vi "Analyze.vi"(8 "error in (no error)":errorcluster, 10 "Image in":T1, 11 "Analyze SHG-AK in":refnum<class "Analyze SHG-AK.lvclass">) -> (0 "error out":errorcluster, 1 "Result":refnum<class "Analyze Results Base.lvclass">, 2 "Image out":T1, 3 "Analyze SHG-AK out":refnum<class "Analyze SHG-AK.lvclass">)   [LabVIEW 2020, in "Analyze.lvlib" / "Analyze SHG-AK.lvclass"]
uses:
  Analyze SHG-AK.lvclass
  C:/POLARIS Programme/POLARIS-AS-3-Cams/Submodules/HIJ Vision/Analyze/Analyze Classes/Analyze BaseClass/Analyze BaseClass/Analyze BaseClass.lvclass
  <vilib>/vision/Image Controls.llb/IMAQ Image.ctl
  Results and Overlays/Results Base/Analyze Results Base.lvclass
  Results and Overlays/Results SHG-AK/Analyze Results SHG-AK.lvclass
  C:/POLARIS Programme/POLARIS-AS-3-Cams/Submodules/HIJ Vision/Analyze/Results and Overlays/Results Base/Analyze Results Base.lvclass
  Analyze Parameter/Analyze Perameter Temporal Calibration/Analyze Parameter Temporal Calibration.lvclass
  C:/POLARIS Programme/POLARIS-AS-3-Cams/Submodules/HIJ Vision/Analyze/Analyze Parameter/Analyze Parameter Base/Analyze Parameter Base.lvclass
  Analyze Parameter/Analyze Perameter Temporal Calibration/Analyze Parameter Temporal Calibration.lvclass/Analyze Parameter Temporal Calibration.ctl
  Results and Overlays/Results SHG-AK/Analyze Results SHG-AK.lvclass/Analyze Results SHG-AK.ctl
  Analyze Parameter/Analyze Perameter Temporal Calibration/Read fs_px.vi
  Results and Overlays/Results SHG-AK/Write Gaussian Fit.vi
  Results and Overlays/Results SHG-AK/Write FWHM .vi
  Results and Overlays/Results SHG-AK/Write X-Values.vi
  Results and Overlays/Results SHG-AK/Write FWHM Gaussfit.vi
  Results and Overlays/Results SHG-AK/Write Y-ROI Averages.vi
  Analyze BaseClass/Analyze BaseClass/Analyze BaseClass.lvclass
  <vilib>/vision/NI_Vision_Development_Module.lvlib
  <vilib>/Analysis/NI_AALPro.lvlib
  Utility/POLARIS Vision utility.lvlib
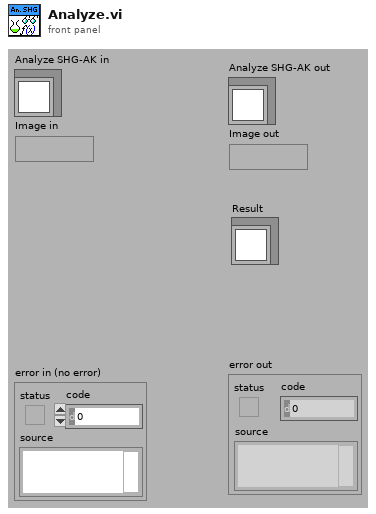
[diagram p1: front panel]
types:
  T1 = typedef "IMAQ Image.ctl" = refnum<image>
  T2 = typedef "ROI Descriptor" = cluster{"Global Rectangle":i32[], "Contours":cluster{"ID":enum32{"External", "Internal"}, "Type":u32, "Coordinates":i32[]}[]}
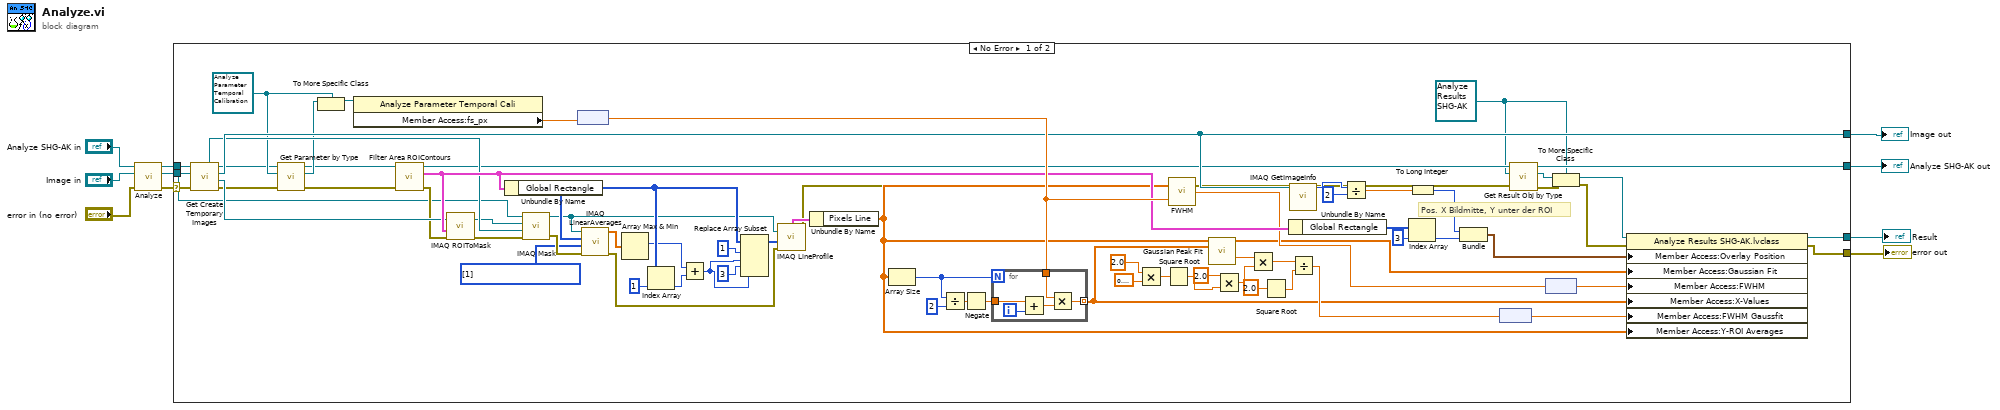
[diagram p0: block diagram]
diagram:
  n1 = call-parent "Analyze.vi"("error in (no error)"="error in (no error)", "Image in"="Image in", "Analyze BaseClass in"="Analyze SHG-AK in") -> ("error out"=w1:errorcluster, "Image out"=w5:T1, "Analyze BaseClass out"=w6:refnum<class "Analyze SHG-AK.lvclass">)  [unwired: 5 in, 1 out]
  n2 = case shown="No Error" w1 {
    selector: w1 -> [w19 w89]
    tunnel: [w67 w88] -> w10
    tunnel: w6 -> [w46 w90]
    tunnel: w5 -> [w45 w88]
    tunnel: [w28 _] -> w4
    tunnel: [w27 w89] -> w3
    tunnel: [w26 w90] -> w2
    frame No Error {
      w17 = refnum<class "Analyze Parameter Temporal Calibration.lvclass"> refnum ("Analyze Parameter Temporal Calibration.lvclass")
      w24 = refnum<class "Analyze Results SHG-AK.lvclass"> refnum ("Analyze Results SHG-AK.lvclass")
      w59 = i32[] [1] items=["X Axis Averages", "Y Axis Averages", "X + Y Axis Averages", "X - Y Axis Averages"] ("Averages")
      # "Pos. X Bildmitte, Y unter der ROI"
      n3 = call-dynamic "Get Create Temporary Images.vi"("error in (no error)"=w19, "Image in"=w45, "Analyze BaseClass in"=w46) -> ("error out"=w14:errorcluster, "image mask"=w65:T1, "work image"=w67:T1, "Analyze BaseClass out"=w15:refnum<class "Analyze SHG-AK.lvclass">, "masked image"=w64:T1)  [unwired: 4 in]
      n4 = call "Get Parameter by Type.vi"("error in (no error)"=w14, "Parameter Type"=w17, "Analyze BaseClass in"=w15) -> ("error out"=w13:errorcluster, "Parameter"=w18:refnum<class "Analyze Parameter Base.lvclass">, "Analyze BaseClass out"=w12:refnum<class "Analyze SHG-AK.lvclass">)  [unwired: 5 in, 1 out]
      n5 = To More Specific Class(target class=w17, reference=w18) -> (specific class reference=w16:refnum<class "Analyze Parameter Temporal Calibration.lvclass">)  [unwired: 1 in, 1 out]
      n6 = property class="Analyze Parameter Temporal Cali"(reference=w16) -> ("Member Access:fs_px"=w11:dbl[unit])  [unwired: 1 in, 2 out]
      n7 = call-dynamic "Filter Area ROIContours.vi"("error in (no error)"=w13, "Analyze BaseClass in"=w12) -> ("error out"=w61:errorcluster, "ROI of Area type"=w66:T2, "Analyze BaseClass out"=w29:refnum<class "Analyze SHG-AK.lvclass">)  [unwired: 7 in]
      n8 = call "IMAQ ROIToMask"("error in (no error)"=w61, "ROI Descriptor"=w66, "Image"=w65) -> ("error out"=w63:errorcluster, "Image Out"=w62:T1)  [unwired: 3 in, 1 out]
      n9 = Unbundle By Name(w66) -> ("Global Rectangle"=w55:i32[])
      n10 = call "IMAQ Mask"("error in (no error)"=w63, "Image Dst"=w64, "Image Mask"=w62, "Image Src"=w45) -> ("error out"=w60:errorcluster, "Image Dst Out"=w50:T1)  [unwired: 1 in]
      n11 = node(w11) -> (w82:dbl)
      n12 = call "IMAQ LinearAverages"("error in (no error)"=w60, "Averages"=w59, "Optional Rectangle"=w55, "Image Src"=w50) -> ("error out"=w48:errorcluster, "Y Axis Averages"=w58:sgl[])  [unwired: 3 in, 3 out]
      n13 = Array Max & Min(array=w58) -> (max index (indices)=w52:i32)  [unwired: 3 out]
      n14 = Index Array(array=w55, index=1) -> (element=w53:i32)
      n15 = Add(x=w52, y=w53) -> (x+y=w51:i32)
      n16 = Replace Array Subset(array=w55, new element #1=w51, index #1=1 ("index"), new element #2=w51, index #2=3 ("index")) -> (w49:i32[])
      n17 = call "IMAQ LineProfile"("error in (no error)"=w48, "Line Coordinates"=w49, "Image"=w50) -> ("error out"=w22:errorcluster, "Line Graph"=w47:cluster{"x0":sgl, "dx":sgl, "Pixels Line":sgl[]})  [unwired: 2 in, 2 out]
      n18 = Unbundle By Name(w47) -> ("Pixels Line"=w42:sgl[])
      n19 = Array Size(array=w42) -> (size(s)=w69:i32)
      n20 = Divide(x=w69, y=2) -> (x/y=w71:dbl)
      n21 = Negate(x=w71) -> (-x=w68:dbl)
      n22 = for {
        N: w69 -> [_]
        tunnel: w68 -> [w86]
        tunnel: [w84] -> w31 mode=indexing
        tunnel: w82 -> [w83]
        i -> [w87]
        n23 = Add(x=w86, y=w87) -> (x+y=w85:dbl)
        n24 = Multiply(x=w83, y=w85) -> (x*y=w84:dbl)
      }
      n25 = Multiply(x=2.0 ("y"), y=0.6931471805599453) -> (x*y=w74:dbl)
      n26 = Square Root(x=w74) -> (sqrt(x)=w75:dbl)
      n27 = call "FWHM.vi"("calibration"=w82, "array"=w42) -> ("FHWM"=w44:dbl)
      n28 = call <vilib>:"Gaussian Peak Fit.vi"("Y"=w42, "X"=w31) -> ("Best Gaussian Fit"=w34:dbl[], "standard deviation"=w81:dbl)  [unwired: 7 in, 5 out]
      n29 = Multiply(x=2.0 ("y"), y=w75) -> (x*y=w76:dbl)
      n30 = Multiply(x=w81, y=w76) -> (x*y=w79:dbl)
      n31 = Square Root(x=2.0) -> (sqrt(x)=w78:dbl)
      n32 = Unbundle By Name(w66) -> ("Global Rectangle"=w41:i32[])
      n33 = call "IMAQ GetImageInfo"("Image"=w67) -> ("X Resolution"=w40:i32)  [unwired: 3 in, 7 out]
      n34 = Divide(x=w79, y=w78) -> (x/y=w43:dbl)
      n35 = Divide(x=w40, y=2) -> (x/y=w38:dbl)
      n36 = To Long Integer(number=w38) -> (32bit integer=w35:i32)
      n37 = Index Array(array=w41, index=3) -> (element=w37:i32)
      n38 = Bundle(w35, w37) -> (w33:cluster{i32, i32})  [unwired: 1 in]
      n39 = node(w43) -> (w32:dbl[unit])
      n40 = call "Get Result Obj by Type.vi"("error in (no error)"=w22, "Parameter Type"=w24, "Analyze BaseClass in"=w29) -> ("error out"=w21:errorcluster, "Parameter"=w25:refnum<class "Analyze Results Base.lvclass">, "Analyze BaseClass out"=w26:refnum<class "Analyze SHG-AK.lvclass">)  [unwired: 5 in, 1 out]
      n41 = node(w44) -> (w30:dbl[unit])
      n42 = To More Specific Class(target class=w24, reference=w25, error in=w21) -> (specific class reference=w23:refnum<class "Analyze Results SHG-AK.lvclass">, error out=w20:errorcluster)
      n43 = property class="Analyze Results SHG-AK.lvclass"(reference=w23, error in=w20, "Member Access:Overlay Position"=w33, "Member Access:Gaussian Fit"=w34, "Member Access:FWHM "=w30, "Member Access:X-Values"=w31, "Member Access:FWHM Gaussfit"=w32, "Member Access:Y-ROI Averages"=w42) -> (reference out=w28:refnum<class "Analyze Results SHG-AK.lvclass">, error out=w27:errorcluster)
    }
    frame Error {
    }
  }
  "error out" <- w3
  "Analyze SHG-AK out" <- w2
  "Image out" <- w10
  "Result" <- w4
